vi "OpenSF.vi"(0 "Port Number":i32=9002) -> (1 "error out":errorcluster, 2 "connection ID":refnum<k5>)   [LabVIEW 2011]
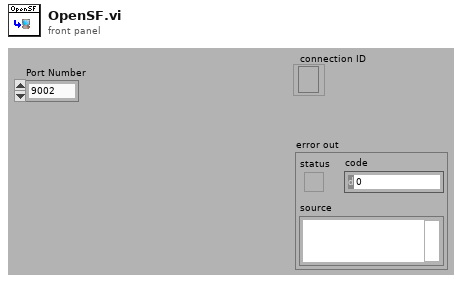
[diagram p1: front panel]
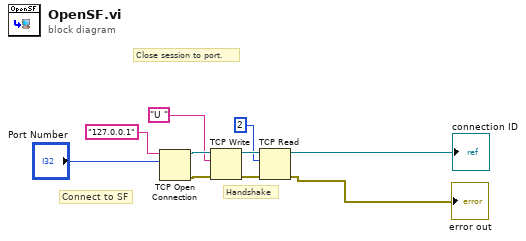
[diagram p0: block diagram]
diagram:
  # "Handshake"
  # "Connect to SF"
  # "Close session to port."
  n1 = TCP Open Connection(address="127.0.0.1", remote port or service name="Port Number") -> (connection ID=w4:refnum<k5>, error out=w3:errorcluster)  [unwired: 3 in]
  n2 = TCP Write(connection ID=w4, data in="U ", error in (no error)=w3) -> (connection ID out=w5:refnum<k5>, error out=w6:errorcluster)  [unwired: 1 in, 1 out]
  n3 = TCP Read(connection ID=w5, bytes to read=2, error in (no error)=w6) -> (connection ID out=→"connection ID":refnum<k5>, error out=→"error out":errorcluster)  [unwired: 2 in, 1 out]
